vi "start.vi"(8 "error in (no error)":errorcluster, 9 "Configuration":string, 10 "model in":refnum<class "IModel.lvclass">, 11 "StandbyState in":refnum<class "StandbyState.lvclass">) -> (0 "error out":errorcluster, 2 "model out":refnum<class "IModel.lvclass">, 3 "StandbyState out":refnum<class "StandbyState.lvclass">)   [LabVIEW 2016, in "States.lvlib" / "StandbyState.lvclass"]
uses:
  StandbyState.lvclass
  IModel/IModel.lvclass
  Typedefs/CommandValue.ctl
  Typedefs/StateValue.ctl
  ts_sallv_exa/DataTypes/logevent_SummaryState.ctl
  Typedefs/EXATypedefs.lvlib
  ComponentTemplateCore/ComponentModel/ComponentModel/ConfigurationFileReader/ConfigurationFileReader.lvclass
  ts_sallv_exa/SALLV_EXA.lvlib
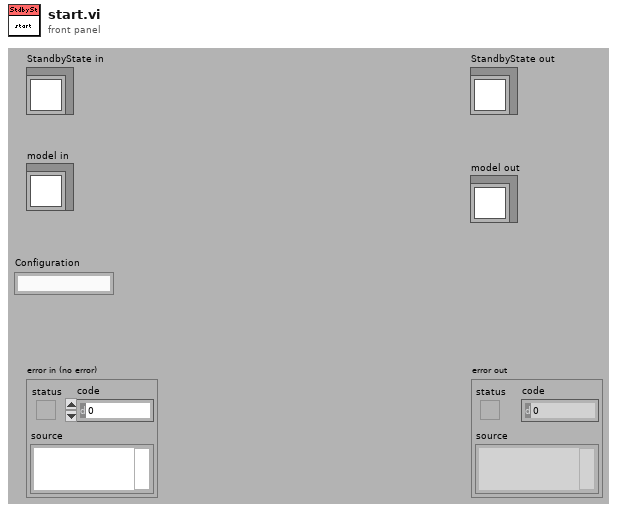
[diagram p1: front panel]
types:
  T1 = typedef "EXATypedefs.lvlib/CommandValue.ctl" = enum16{"ClearError", "Disable", "Enable", "Exit", "GoToStandby", "OnHeartbeat", "OnIncomingMessagingError", "OnInterrupt", "Start"}
  T2 = typedef "SALLV_EXA.lvlib/logevent_SummaryState.ctl" = cluster{"summaryState":enum16{"", " OfflineState", "StandbyState", "DisabledState", "EnabledState", "FaultState"}, "priority":i32}
  T3 = typedef "EXATypedefs.lvlib/StateValue.ctl" = enum16{"", " DisabledState", "EnabledState", "FaultState", "OfflineState", "StandbyState"}
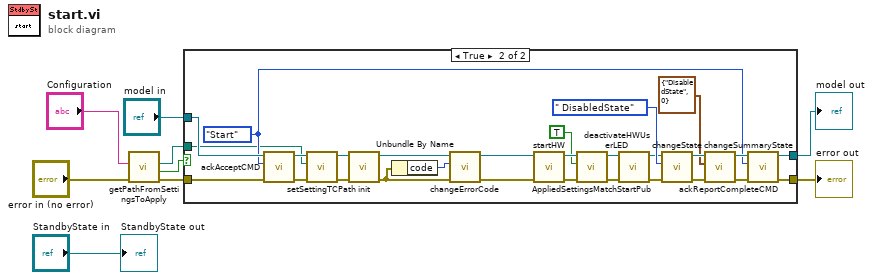
[diagram p0: block diagram]
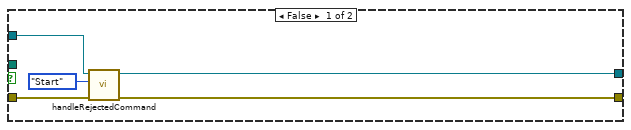
[diagram p2: hidden frame]
diagram:
  n1 = call "getPathFromSettingsToApply.vi"("error in (no error)"="error in (no error)", "SettingToApply"="Configuration") -> ("error out"=w3:errorcluster, "labelExist?"=w2:bool, "SettingsPath"=w1:path)  [unwired: 6 in, 1 out]
  n2 = case shown="True" w2 {
    tunnel: "model in" -> [w12 w34]
    tunnel: [w13 w33] -> w7
    tunnel: [w11 w30] -> w6
    tunnel: w3 -> [w14 w20]
    tunnel: w1 -> [_ w18]
    frame False {
      n3 = call-dynamic "handleRejectedCommand.vi"("error in (no error)"=w14, "CommandValue"=CommandValue."Start", "IModel in"=w12) -> ("error out"=w13:errorcluster, "IModel out"=w11:refnum<class "IModel.lvclass">)  [unwired: 7 in]
    }
    frame True {
      w29 = CommandValue."Start" ("CommandValue")
      n4 = call-dynamic "ackAcceptCMD.vi"("error in (no error)"=w20, "CommandValue"=w29, "IModel in"=w34) -> ("error out"=w19:errorcluster, "IModel out"=w21:refnum<class "IModel.lvclass">)  [unwired: 7 in]
      n5 = call-dynamic "setSettingTCPath.vi"("error in (no error)"=w19, "Path"=w18, "IModel in"=w21) -> ("error out"=w23:errorcluster, "IModel out"=w22:refnum<class "IModel.lvclass">)  [unwired: 7 in]
      n6 = call-dynamic "init.vi"("error in (no error)"=w23, "IModel in"=w22) -> ("error out"=w37:errorcluster, "IModel out"=w38:refnum<class "IModel.lvclass">)  [unwired: 8 in]
      n7 = Unbundle By Name(w37) -> ("code"=w39:i32)
      n8 = call-dynamic "changeErrorCode.vi"("error in (no error)"=w37, "error.code"=w39, "IModel in"=w38) -> ("error out"=w16:errorcluster, "IModel out"=w17:refnum<class "IModel.lvclass">)  [unwired: 7 in]
      n9 = call-dynamic "startHW.vi"("error in (no error)"=w16, "IModel in"=w17) -> ("error out"=w28:errorcluster, "IModel out"=w25:refnum<class "IModel.lvclass">)  [unwired: 8 in]
      n10 = call-dynamic "AppliedSettingsMatchStartPub.vi"("error in (no error)"=w28, "Applied?"=TRUE, "IModel in"=w25) -> ("error out"=w27:errorcluster, "IModel out"=w26:refnum<class "IModel.lvclass">)  [unwired: 7 in]
      n11 = call-dynamic "deactivateHWUserLED.vi"("error in (no error)"=w27, "IModel in"=w26) -> ("error out"=w35:errorcluster, "IModel out"=w36:refnum<class "IModel.lvclass">)  [unwired: 8 in]
      n12 = call-dynamic "changeState.vi"("error in (no error)"=w35, "newState"=StateValue." DisabledState" ("StateValue"), "IModel in"=w36) -> ("error out"=w40:errorcluster, "IModel out"=w41:refnum<class "IModel.lvclass">)  [unwired: 7 in]
      n13 = call-dynamic "changeSummaryState.vi"("error in (no error)"=w40, "logevent_SummaryState"=T2 {"summaryState"=enum."DisabledState", "priority"=0}, "IModel in"=w41) -> ("error out"=w32:errorcluster, "IModel out"=w31:refnum<class "IModel.lvclass">)  [unwired: 7 in]
      n14 = call-dynamic "ackReportCompleteCMD.vi"("error in (no error)"=w32, "CommandValue"=w29, "IModel in"=w31) -> ("error out"=w33:errorcluster, "IModel out"=w30:refnum<class "IModel.lvclass">)  [unwired: 7 in]
    }
  }
  "error out" <- w7
  "model out" <- w6
  "StandbyState out" <- "StandbyState in"
